vi "ProcessName.vi"() -> (1 "process name":string="EmsaAudio")   [LabVIEW 2017, in "EmsaAudio.lvlib"]
uses:
  <vilib>/addons/InsightCM/Devices/Shared/Emsa/EmsaAudio/EmsaAudio.lvlib
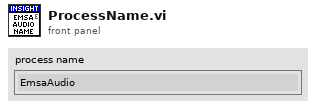
[diagram p1: front panel]
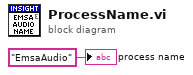
[diagram p0: block diagram]
diagram:
  "process name" <- "EmsaAudio" ("ProcessName")
